vi "Istwerte verarbeiten UsrVal.vi"(8 "error in (no error)":errorcluster caption="Fehler (Eingang, kein Fehler)", 10 "Istwerte":u16[](array[numeric]), 11 "Steuerung PNS Eingang":refnum<class "Steuerung PNS.lvclass">) -> (0 "error out":errorcluster caption="Fehler (Ausgang)", 3 "Steuerung PNS Ausgang":refnum<class "Steuerung PNS.lvclass">)   [LabVIEW 2020, in "Steuerung PNS.lvclass"]
uses:
  Steuerung PNS.lvclass
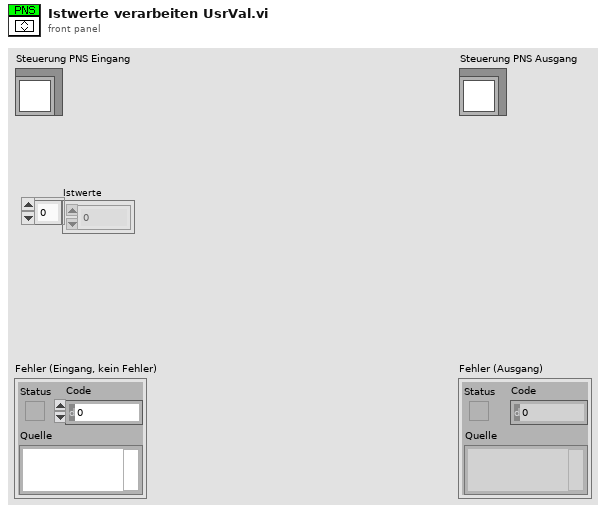
[diagram p1: front panel]
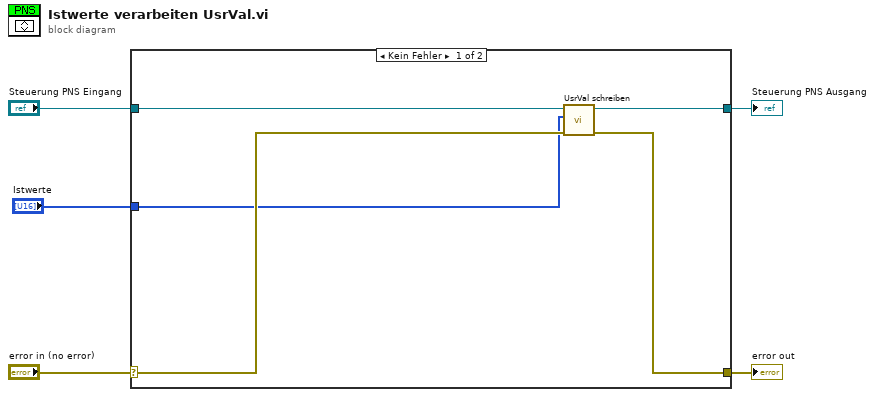
[diagram p0: block diagram]
diagram:
  n1 = case shown="Kein Fehler" "error in (no error)" {
    selector: "error in (no error)" -> [w8 w12]
    tunnel: [w7 w12] -> w4
    tunnel: [w9 w11] -> w2
    tunnel: "Steuerung PNS Eingang" -> [w10 w11]
    tunnel: "Istwerte" -> [w6 _]
    frame No Error {
      n2 = call-dynamic "UsrVal schreiben.vi"("error in (no error)"=w8, "UsrVal"=w6, "Steuerung PNS (Eingang)"=w10) -> ("error out"=w7:errorcluster, "Steuerung PNS (Ausgang)"=w9:refnum<class "Steuerung PNS.lvclass">)  [unwired: 7 in]
    }
    frame Error {
    }
  }
  "error out" <- w4
  "Steuerung PNS Ausgang" <- w2
